vi "ConfigureStartupAnalysis.vi"(8 "error in (no error)":errorcluster) -> (0 "error out":errorcluster, 3 "groups for startup measurement":T1, 5 "valid config?":bool)   [LabVIEW 2017, in "McsaStartupAnalysis.lvlib"]
uses:
  <vilib>/addons/InsightCM/Devices/Shared/Mcsa/McsaStartupAnalysis/McsaStartupAnalysis.lvlib
  <vilib>/addons/InsightCM/Devices/Shared/Mcsa/McsaStartupAnalysis/controls/Config.ctl
  <vilib>/addons/InsightCM/Devices/Shared/Mcsa/McsaStartupAnalysis/controls/Group.ctl
  <vilib>/addons/InsightCM/Devices/Shared/Mcsa/McsaStartupAnalysis/controls/ChannelForStartup.ctl
  <vilib>/addons/InsightCM/Devices/Shared/Mcsa/McsaStartupAnalysis/controls/StartupFeature.ctl
  <vilib>/addons/InsightCM/Devices/Shared/Mcsa/McsaStartupAnalysis/controls/MotorInfo.ctl
  <vilib>/addons/InsightCM/MessageBus/Base/controls/R2_DeviceModel.ctl
  <vilib>/addons/InsightCM/MessageBus/Base/controls/R2_Device.ctl
  <vilib>/addons/InsightCM/MessageBus/Base/controls/KeyValuePair.ctl
  <vilib>/addons/InsightCM/MessageBus/Base/controls/DeviceState.ctl
  <vilib>/addons/InsightCM/MessageBus/Base/controls/R2_DataGroup.ctl
  <vilib>/addons/InsightCM/MessageBus/Base/controls/OperatingState.ctl
  <vilib>/addons/InsightCM/MessageBus/Base/controls/Trigger.ctl
  <vilib>/addons/InsightCM/MessageBus/Base/controls/Condition.ctl
  <vilib>/addons/InsightCM/MessageBus/Base/controls/BurstModeTrigger.ctl
  <vilib>/addons/InsightCM/MessageBus/Base/controls/R2_Channel.ctl
  <vilib>/addons/InsightCM/MessageBus/Base/controls/Metric.ctl
  <vilib>/addons/InsightCM/MessageBus/Base/controls/Tag.ctl
  <vilib>/addons/InsightCM/Utilities/GlobalConfiguration/GlobalConfiguration.lvlib
  <vilib>/addons/InsightCM/Utilities/DeviceModelHelpers/DeviceModelHelpers.lvlib
  <vilib>/addons/InsightCM/Utilities/Analysis/Shared/AnalysisHelper.lvlib
  <vilib>/addons/InsightCM/Devices/Shared/Mcsa/McsaVirtualChannel/McsaVirtualChannel.lvlib
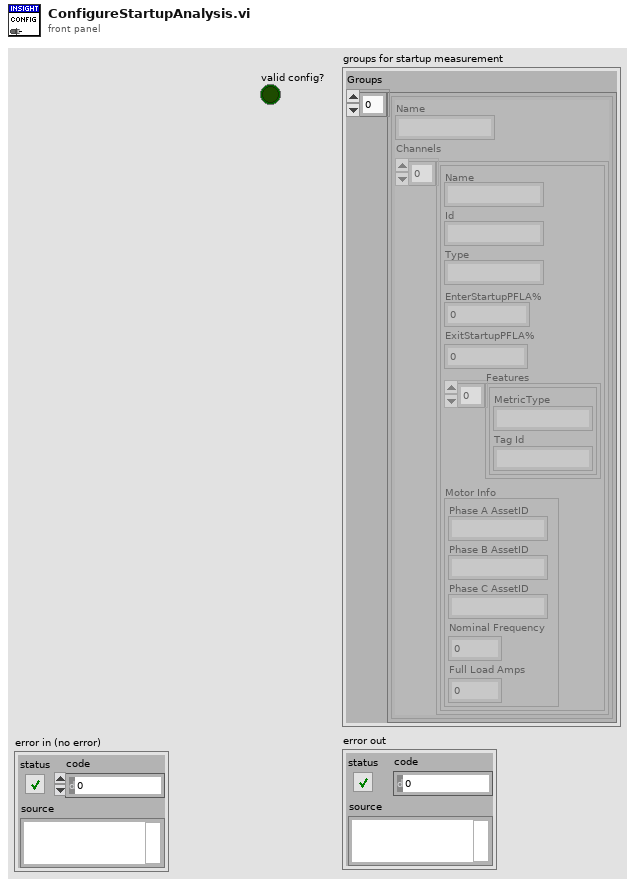
[diagram p1: front panel]
types:
  T1 = typedef "McsaStartupAnalysis.lvlib/Config.ctl" = cluster{"Groups":T2[]}
  T2 = typedef "McsaStartupAnalysis.lvlib/Group.ctl" = cluster{"Name":string, "Channels":T3[]}
  T3 = typedef "McsaStartupAnalysis.lvlib/ChannelForStartup.ctl" = cluster{"Name":string, "Id":string, "Type":string, "EnterStartupPFLA%":dbl, "ExitStartupPFLA%":dbl, "Features":T4[], "Motor Info":T5}
  T4 = typedef "McsaStartupAnalysis.lvlib/StartupFeature.ctl" = cluster{"MetricType":string, "Tag Id":string}
  T5 = typedef "McsaStartupAnalysis.lvlib/MotorInfo.ctl" = cluster{"Phase A AssetID":string, "Phase B AssetID":string, "Phase C AssetID":string, "Nominal Frequency":dbl, "Full Load Amps":dbl}
  T6 = typedef "R2_DeviceModel.ctl" = cluster{"Device":T7, "Channels":T15[], "Tags":T17[]}
  T7 = typedef "R2_Device.ctl" = cluster{"Id":string, "Name":string, "DeviceType":string, "HardwareName":string, "IpAddress":string, "HardwareInfo":T8[], "ApplicationType":string, "ApplicationVersion":string, "EquipmentIds":string[], "ConfigurationVersion":string, "State":T9, "Properties":T8[], "DataGroups":T10[], "BurstModeTrigger":T14}
  T8 = typedef "KeyValuePair.ctl" = cluster{"Key":string, "Value":string}
  T9 = typedef "DeviceState.ctl" = cluster{"Disabled":bool}
  T10 = typedef "R2_DataGroup.ctl" = cluster{"Name":string, "OperatingStates":T11[], "Properties":T8[], "EquipmentIds":string[], "AssetNodeId":string}
  T11 = typedef "OperatingState.ctl" = cluster{"Name":string, "Properties":T8[], "Triggers":T12[]}
  T12 = typedef "Trigger.ctl" = cluster{"Type":string, "Expression":string, "Conditions":T13[]}
  T13 = typedef "Condition.ctl" = cluster{"Source":string, "Type":string, "Operator":string, "CompareTo":string, "DwellSeconds":dbl}
  T14 = typedef "BurstModeTrigger.ctl" = cluster{"Trigger":T12, "SampleRate":string, "AcquisitionLength":string}
  T15 = typedef "R2_Channel.ctl" = cluster{"Id":string, "DeviceId":string, "Name":string, "ChannelType":string, "HardwareKey":string, "HardwareChannel":string, "DataGroup":string, "Keywords":string[], "EquipmentIds":string[], "Properties":T8[], "Metrics":T16[], "AssetNodeId":string, "MeasType":string, "AssetName":string}
  T16 = typedef "Metric.ctl" = cluster{"Id":string, "Name":string, "Unit":string, "Properties":T8[], "MetricDefinitionInstanceId":string}
  T17 = typedef "Tag.ctl" = cluster{"Id":string, "Path":string, "Name":string, "Datatype":string, "Props":T8[], "Keywords":string[]}
  T18 = typedef "MetricDefinitionInstance.ctl" = cluster{"Id":string, "MetricType":string, "Name":string, "Properties":T8[], "HighRate":bool}
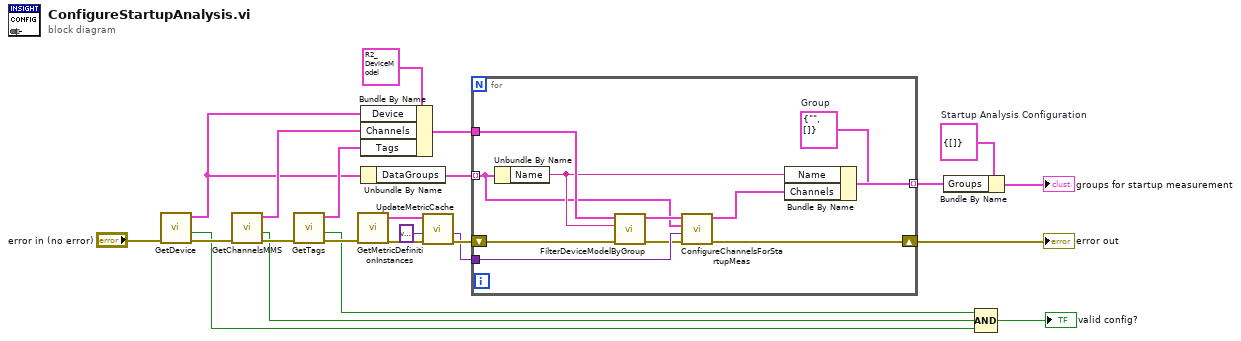
[diagram p0: block diagram]
diagram:
  w7 = T1 {"Groups"=[]}  # Startup Analysis Configuration
  n1 = call <vilib>:"GetDevice.vi"("error in (no error)"="error in (no error)") -> ("error out"=w9:errorcluster, "found"=w3:bool, "device configuration"=w1:T7)  [unwired: 8 in]
  n2 = call <vilib>:"GetChannelsMMS.vi"("error in (no error)"=w9) -> ("error out"=w23:errorcluster, "found"=w4:bool, "MMS Channels"=w10:T15[])  [unwired: 6 in, 2 out]
  n3 = call <vilib>:"GetTags.vi"("error in (no error)"=w23) -> ("error out"=w21:errorcluster, "found"=w5:bool, "tags"=w19:T17[])  [unwired: 8 in]
  n4 = call <vilib>:"GetMetricDefinitionInstances.vi"("error in (no error)"=w21) -> ("error out"=w18:errorcluster, "metrics"=w16:T18[])  [unwired: 8 in, 1 out]
  n5 = Bundle By Name(cluster=T6 {"Device"={"Id"="", "Name"="", "DeviceType"="", "HardwareName"="", "IpAddress"="", "HardwareInfo"=[], "ApplicationType"="", "ApplicationVersion"="", "EquipmentIds"=[], "ConfigurationVersion"="", "State"={"Disabled"=FALSE}, "Properties"=[], "DataGroups"=[], "BurstModeTrigger"={"Trigger"={"Type"="", "Expression"="", "Conditions"=[]}, "SampleRate"="", "AcquisitionLength"=""}}, "Channels"=[], "Tags"=[]} ("Asset Manager Device Model"), "Device"=w1, "Channels"=w10, "Tags"=w19) -> (w11:T6)
  n6 = Unbundle By Name(w1) -> ("DataGroups"=w13:T10[])
  n7 = call <vilib>:"UpdateMetricCache.vi"("error in (no error)"=w18, "Metrics"=variant, "MetricDefinitionInstances"=w16) -> ("error out"=w17:errorcluster, "Metrics out"=w15:variant)  [unwired: 7 in]
  n8 = for {
    tunnel: w15 -> [w34]
    tunnel: w11 -> [w29]
    shift-right: [w28] -> w12
    shift-left: w17 -> [w31]
    tunnel: [w33] -> w8 mode=indexing
    tunnel: w13 -> [w24] mode=indexing
    w27 = T2 {"Name"="", "Channels"=[]}  # Group
    n9 = Unbundle By Name(w24) -> ("Name"=w25:string)
    n10 = call <vilib>:"FilterDeviceModelByGroup.vi"("error in (no error)"=w31, "group"=w25, "device model"=w29) -> ("error out"=w30:errorcluster, "device model (channels filtered by group)"=w32:T6)  [unwired: 7 in]
    n11 = call <vilib>:"ConfigureChannelsForStartupMeas.vi"("error in (no error)"=w30, "metric cache"=w34, "DataGroup"=w24, "device"=w32) -> ("error out"=w28:errorcluster, "valid channels for startup measurement"=w26:T3[])  [unwired: 6 in]
    n12 = Bundle By Name(cluster=w27, "Name"=w25, "Channels"=w26) -> (w33:T2)
  }
  "error out" <- w12
  n13 = Bundle By Name(cluster=w7, "Groups"=w8) -> (→"groups for startup measurement":T1)
  n14 = Compound Arithmetic op=AND(w5, w4, w3) -> (→"valid config?":bool)
